vi "Map RTD.vi"(6 "Signal List Keys":T1, 8 "error in":errorcluster, 10 "RTD_String":string[](array[string]), 11 "PRM in":refnum<class "PRM.lvclass">) -> (0 "error out":errorcluster, 3 "PRM out":refnum<class "PRM.lvclass">)   [LabVIEW 2019, in "PRM.lvlib" / "PRM.lvclass"]
uses:
  Library/PRM.lvclass
  Custom Controls/Signal List Keys.ctl
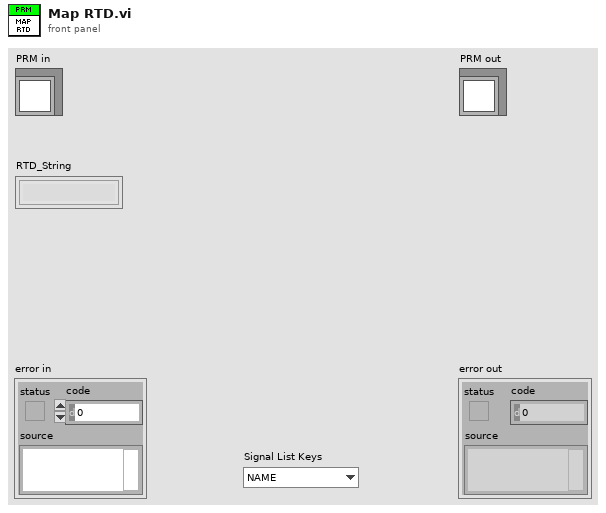
[diagram p1: front panel]
types:
  T1 = typedef "PRM.lvlib/PRM.lvclass/Signal List Keys.ctl" = enum16{"NAME", "MAX", "MIN", "RTD_A", "RTD_B", "RTD_C", "RTD_R0"}
  T2 = typedef "PRM.lvlib/PRM.lvclass/RTD Parameters.ctl" = cluster{"A":dbl, "B":dbl, "C":dbl, "R0":dbl}
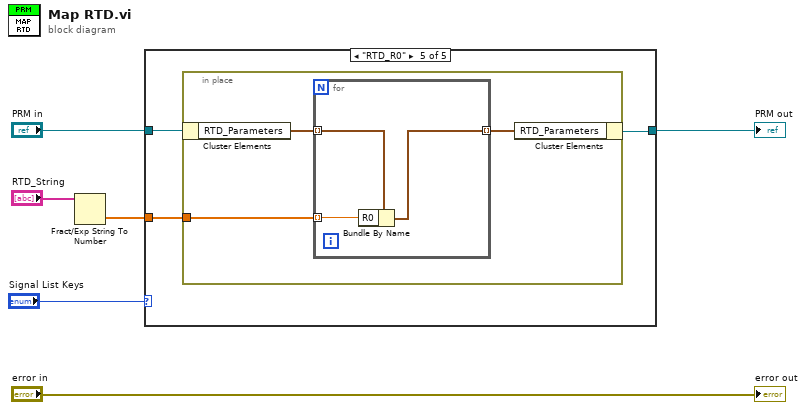
[diagram p0: block diagram]
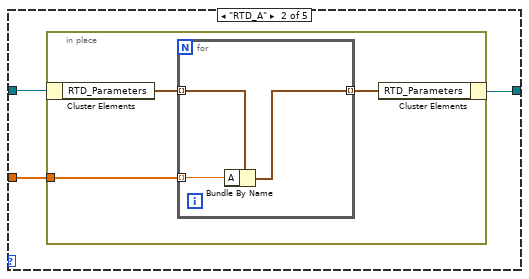
[diagram p3: hidden frame]
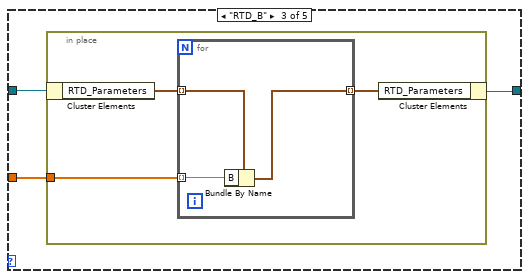
[diagram p4: hidden frame]
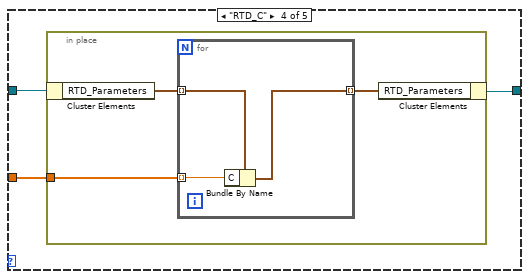
[diagram p5: hidden frame]
diagram:
  n1 = Fract/Exp String To Number(string="RTD_String") -> (number=w1:dbl[])  [unwired: 3 in, 1 out]
  n2 = case shown="\"RTD_R0\"" "Signal List Keys" {
    tunnel: "PRM in" -> [w7 w10 w19 w28 w37]
    tunnel: [w7 w9 w18 w27 w36] -> w3
    tunnel: w1 -> [_ w8 w17 w26 w35]
    frame "NAME", Default {
    }
    frame "RTD_A" {
      n3 = in-place {
        in-place-border: w8 -> [w12]
        n4 = in-place-cluster #1(w10) -> ("RTD_Parameters"=w13:T2[])
        n5 = for {
          tunnel: w13 -> [w16] mode=indexing
          tunnel: w12 -> [w15] mode=indexing
          tunnel: [w14] -> w11 mode=indexing
          n6 = Bundle By Name(cluster=w16, "A"=w15) -> (w14:T2)
        }
        n7 = in-place-cluster #1("RTD_Parameters"=w11) -> (w9:refnum<class "PRM.lvclass">)
      }
    }
    frame "RTD_B" {
      n8 = in-place {
        in-place-border: w17 -> [w21]
        n9 = in-place-cluster #2(w19) -> ("RTD_Parameters"=w22:T2[])
        n10 = for {
          tunnel: w22 -> [w25] mode=indexing
          tunnel: w21 -> [w24] mode=indexing
          tunnel: [w23] -> w20 mode=indexing
          n11 = Bundle By Name(cluster=w25, "B"=w24) -> (w23:T2)
        }
        n12 = in-place-cluster #2("RTD_Parameters"=w20) -> (w18:refnum<class "PRM.lvclass">)
      }
    }
    frame "RTD_C" {
      n13 = in-place {
        in-place-border: w26 -> [w30]
        n14 = in-place-cluster #3(w28) -> ("RTD_Parameters"=w31:T2[])
        n15 = for {
          tunnel: w31 -> [w34] mode=indexing
          tunnel: w30 -> [w33] mode=indexing
          tunnel: [w32] -> w29 mode=indexing
          n16 = Bundle By Name(cluster=w34, "C"=w33) -> (w32:T2)
        }
        n17 = in-place-cluster #3("RTD_Parameters"=w29) -> (w27:refnum<class "PRM.lvclass">)
      }
    }
    frame "RTD_R0" {
      n18 = in-place {
        in-place-border: w35 -> [w39]
        n19 = in-place-cluster #4(w37) -> ("RTD_Parameters"=w40:T2[])
        n20 = for {
          tunnel: w40 -> [w43] mode=indexing
          tunnel: w39 -> [w42] mode=indexing
          tunnel: [w41] -> w38 mode=indexing
          n21 = Bundle By Name(cluster=w43, "R0"=w42) -> (w41:T2)
        }
        n22 = in-place-cluster #4("RTD_Parameters"=w38) -> (w36:refnum<class "PRM.lvclass">)
      }
    }
  }
  "PRM out" <- w3
  "error out" <- "error in"
